vi "Dashboard2013.vi"() -> ()   [LabVIEW 2015]
uses:
  <vilib>/Utility/config.llb/NI_LVConfig.lvlib
  <vilib>/Utility/config.llb/Write Key (I32).vi
  globals/Angle.vi
  <vilib>/FTP/NI_FTP.lvlib
  <vilib>/vision/NI_Vision_Development_Module.lvlib
  <vilib>/Platform/browser.llb/Open URL in Default Browser (string).vi
  <vilib>/event_ctls.llb/eventvkey.ctl
  <vilib>/Utility/config.llb/Write Key (String).vi
  <vilib>/Utility/config.llb/Read Key (Double).vi
  <vilib>/Utility/config.llb/Write Key (Double).vi
  typeDefs/targetVariables.ctl
panel:
  in  "Filename":string="filename"
  in  "CaptureScreen":bool caption="OK Button"
  out "standard output":string
  in  "Tab Control":enum32{"Main", "Diagnostic"}(tab)
  in  "Viewer":enum32{"Camera", "Variables", "Files", "Misc"}(tab)
  out "Shoot Adjust":i8(slide) scale=-100.0..100.0 scale format="%4d"
  out "Image Error Message":string="Timeout in Camera Communications"
  out "Speed":cluster{dbl, dbl}(knob)={0.0, 3409.0831639982152} scale=2500.0..4300.0
  out "Frisbees":i16 format="%1.0f"
  out "Angle to Center":dbl format="%#_3g"
  out "Range to Center":dbl format="%-#3_3g"
  in  "Low Camera Settings":T1={"Frate Rate"=30, "Compression"=30, "Size"=1} {"Frate Rate" scale=1.0..30.0; "Size" items=["640x480", "320x240", "160x120"]}
  out "L Mbps":dbl format="%#.1g"
  in  "Low Cam Conf":bool
  out "BW":bool
  out "L_FPS":dbl format="%#.1g"
  out "Low Camera Image":T2(plugin-control) caption="Camera Image"
  in  "High Cam Conf":bool
  out "In Range":bool=TRUE
  out "Pre Hopper Time":dbl
  out "Pre-Jam":bool
  out "Batt Voltage":dbl
  in  "y":bool
  out "Tree":string(tree)
  in  "Open Auto Commands Doc":bool
  in  "Edit Vision Distance Table CSV":bool
  in  "Edit Autonomous CSV":bool
  in  "Transfer Vision Distance Table  to cRIO":bool
  in  "working directory":path=path "C:/BB/2013/Programming/Beachbot2013Dashboard"
  out "standard output":string
  in  "Transfer Autonomous CSV to cRIO":bool
  in  "Transfer INI From cRIO":bool
  in  "upper limit":dbl=20.0
  in  "lower limit":dbl=19.0
  in  "Dashboard Tab":T3(tab)
  in  "AutoWait":u16 caption="Autonomous Delay (Seconds)" format="%#7.0f"
  out "Battery Value":dbl(slide) scale=0.0..14.0 scale format="%#_2e"
  out "Battery":sgl(graph)
  out "Robot IP":string
  in  "Autonomous\nMode":u16(ring)
  in  "Number":dbl caption="rightDriveP"
  in  "Preferences Tree":string(tree)
  in  "Save":bool
  in  "On/Off":bool caption="~S A V E~"
  in  "String":string caption="Strings"
  in  "Slider":dbl(slide) scale=0.0..100.0 scale format="%#_3g"
  in  "What is this?":bool
  in  "Test Name":u16(ring) items=["Select the test to run...", "Example Test", "-------------------------------", "List of tests is built in robot code.", "Replace with your own automated tests."]
  in  "Test Tree":string(tree)
  in  "Motor":cluster{"Value":dbl, "Enable":bool} {"Value" scale=-1.0..1.0 scale format="%#_3g"}
  out "Progress":T4 {"Test Progress" scale=0.0..100.0}
  in  "Rev/Fwd":cluster{"Forward":bool, "Reverse":bool}
  in  "Ring":u16(ring) items=["Auto", "Fixed indoor", "Fixed outdoor 1", "Fixed outdoor 2", "Fixed fluorescent 1", "Fixed fluorescent 2", "Hold current"]
  in  "Listbox":i32(listbox)
  in  "BCG Low":T5={"Brightness"=212.0, "Contrast"=59.7, "Gamma"=0.64}
  out "Mode":T6(ring)=enum."Auto Disabled"
  in  "Alignment":i32=50
  in  "Targeting":i32=37
  out "Low Camera IP":string
  out "Target Info":T7(array[cluster]) {"Center Position"."X" format="%#_3g"; "Center Position"."Y" format="%#_3g"}
  in  "Camera view angle":dbl[](array[numeric])=[48.0, 43.5]
  out "Processed Image":T2(plugin-control)
  in  "Low Dilate_its":i32=11
  in  "Low Erode_its":i32=12
  in  "Low Brightness":i32=50
  out "Values":T8
  in  "Manual Video IP":bool
  out "Camera Image Diag":T2(plugin-control) caption="Camera Image"
  # "Shooting Range Setting"
  # "Audio Settings"
  # "Robot IP:"
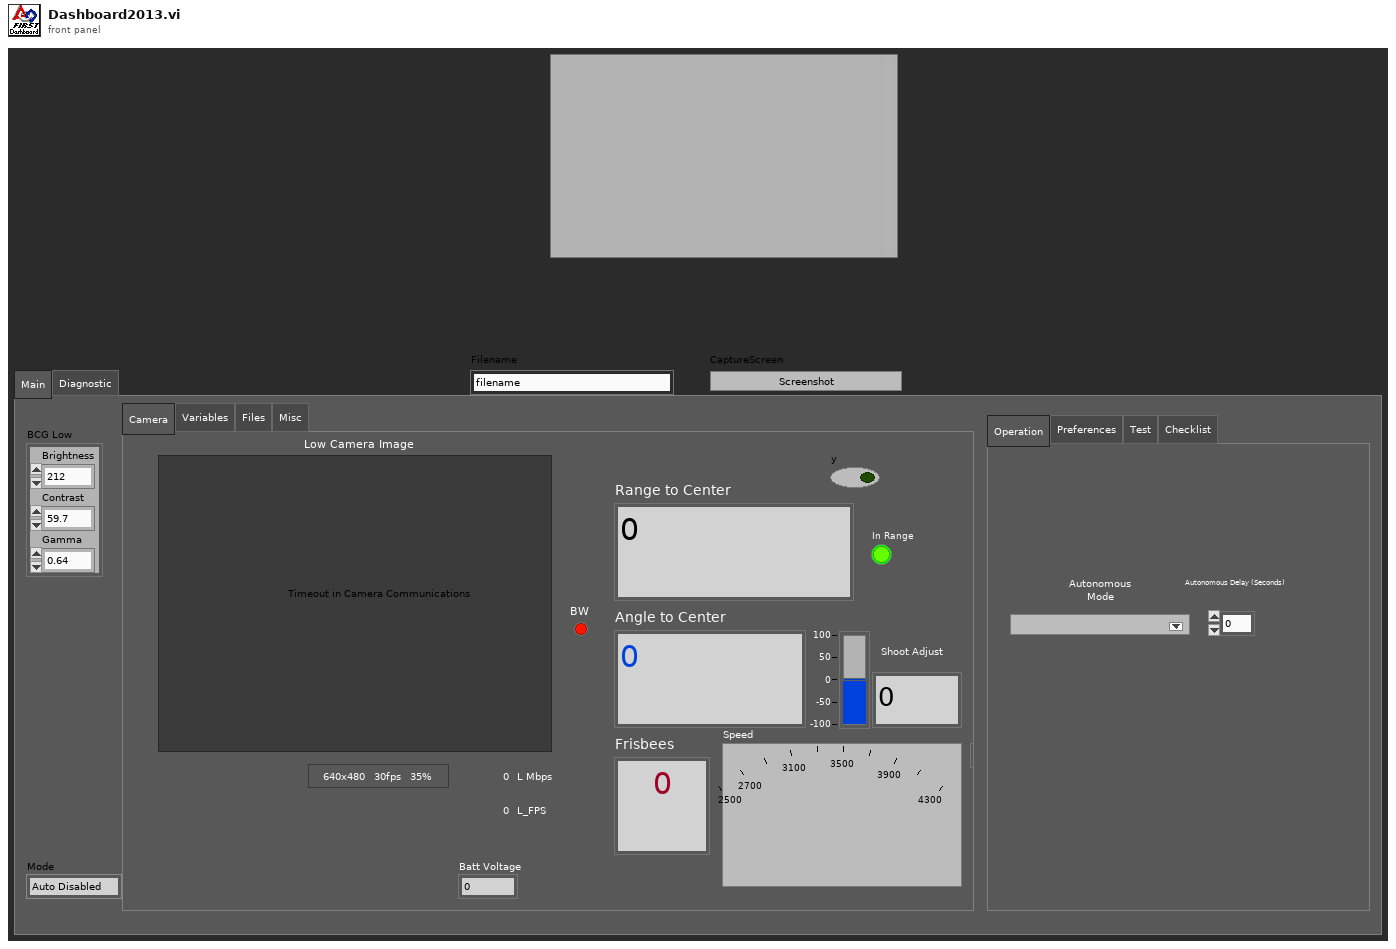
[diagram p1: front panel]
types:
  T1 = cluster{"Frate Rate":i32, "Compression":i32, "Size":u16}
  T2 = typedef "IMAQ Image.ctl" = refnum<image>
  T3 = enum32{"Operation", "Preferences", "Test", "Checklist"}
  T4 = cluster{"Test Progress":u8, "Test Progress Text":string}
  T5 = cluster{"Brightness":sgl, "Contrast":sgl, "Gamma":sgl}
  T6 = enum8{"Tele-Op Disabled", "Tele-Op Enabled", "Auto Disabled", "Auto Enabled", "Test Disabled", "Test Enabled", ""}
  T7 = cluster{"Center Position":cluster{"X":dbl, "Y":dbl}, "Distance":dbl, "targetType":enum16{"Center", "Side", "Vertical"}}[]
  T8 = typedef "targetVariables.ctl" = cluster{"distanceToCenter":dbl, "angleToCenter":dbl, "angleToLeft":dbl, "distanceToLeft":dbl, "angleToRight":dbl, "distanceToRight":dbl, "centerAge":dbl, "leftAge":dbl, "rightAge":dbl}
  T9 = typedef "Image Type" = u32
  T10 = typedef "Sound Output Task ID.ctl" = u32
  T11 = typedef "SkeletonTrackState.ctl" = enum32{"NotTracked", "PositionOnly", "Tracked"}
  T12 = cluster{"TrackingState":u8[], "Position":cluster{"x":sgl, "y":sgl, "z":sgl}, cluster{"x":sgl, "y":sgl, "z":sgl, sgl}[], "TrackState":T11}
  T13 = cluster{cluster{"ScaledToPercentRange":dbl, "ScaledToPercentRange":dbl, "ScaledToPercentRange":dbl}, cluster{bool, bool, bool}}[]
  T14 = cluster{cluster{"ScaledToPercentRange":dbl, "ScaledToPercentRange":dbl, "ScaledToPercentRange":dbl}, cluster{bool, bool, bool}}
  T15 = typedef "LVRectTypeDef.ctl" = cluster{"Left":i16, "Top":i16, "Right":i16, "Bottom":i16}
  T16 = cluster{"Competition mode":bool, "Robot Link":bool, "Autonomous":bool, "Enabled":bool, "E-Stop":bool, "Simulated":bool, "TestMode":bool, "Docked Window":bool}
  T17 = typedef "NI_LVConfig.lvlib/Config Data RefNum.ctl" = refnum<k1>
  T18 = typedef "eventvkey.ctl" = enum16{"ASCII", "Enter", "Return", "Shift", "Ctrl", "Alt", "Cmd", "Opt", "Caps", "NumLock", "Clear", "Break", "Up", "Down", "Left", "Right", "Insert", "Delete", "Home", "End", "PageUp", "PageDown", "Escape", "Help", "Pause", "ScrollLock", "F1", "F2", "F3", "F4", "F5", "F6", "F7", "F8", "F9", "F10", "F11", "F12", "F13", "F14", "F15", "F16", "F17", "F18", "F19", "F20", "F21", "F22", "F23", "F24", "Play", "VolumeUp", "VolumeDown", "Mute", "Two Byte Char"}
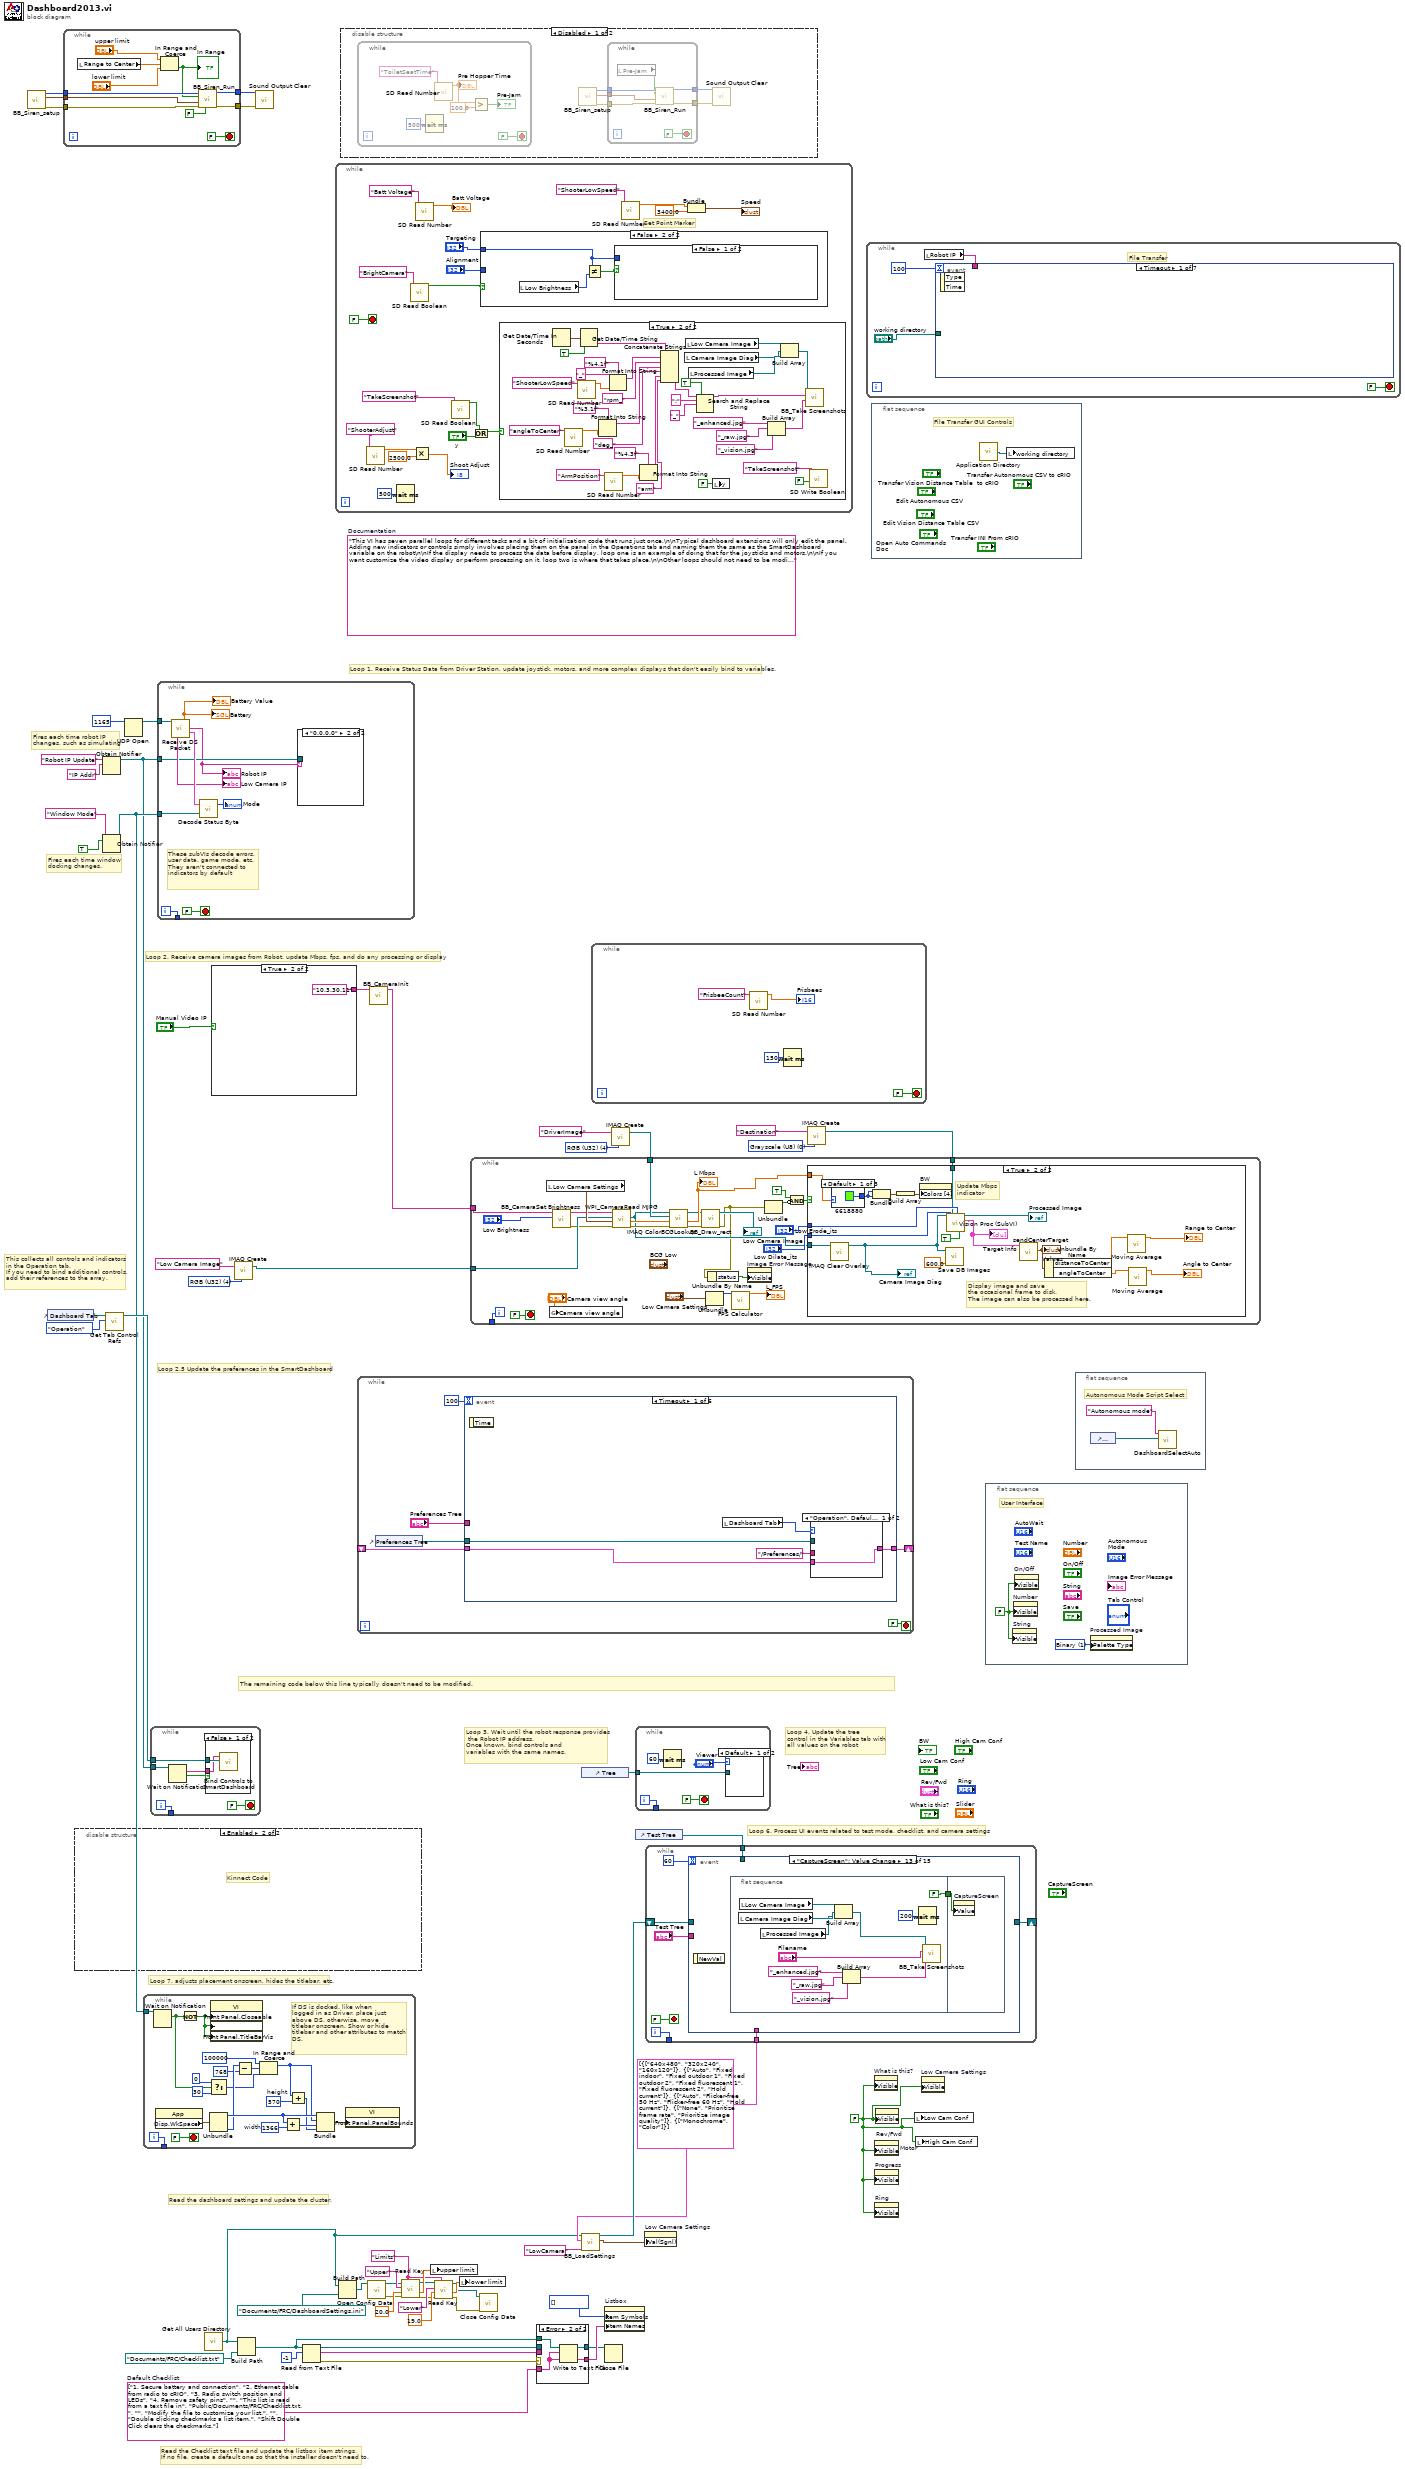
[diagram p0: block diagram]
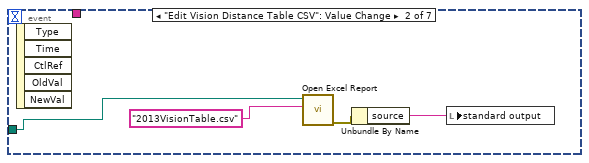
[diagram p2: hidden frame]
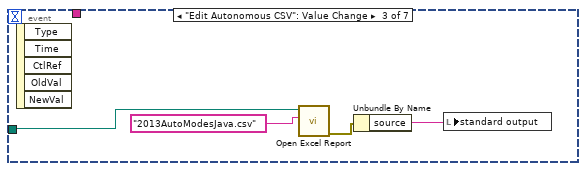
[diagram p3: hidden frame]
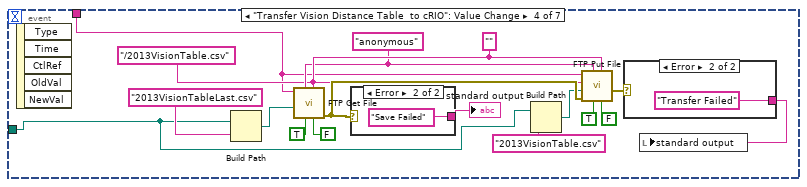
[diagram p4: hidden frame]
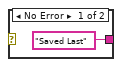
[diagram p5: hidden frame]
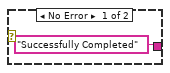
[diagram p6: hidden frame]
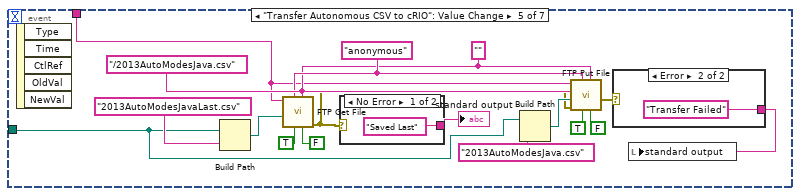
[diagram p7: hidden frame]
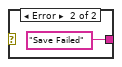
[diagram p8: hidden frame]
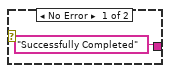
[diagram p9: hidden frame]
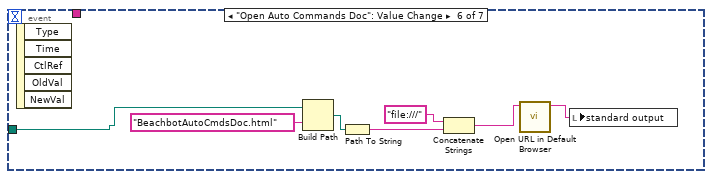
[diagram p10: hidden frame]
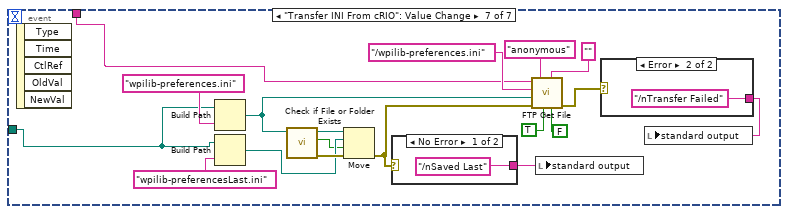
[diagram p11: hidden frame]
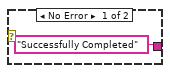
[diagram p12: hidden frame]
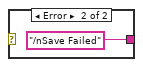
[diagram p13: hidden frame]
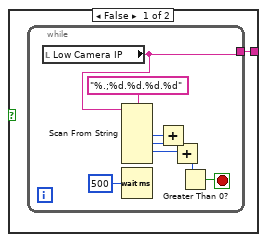
[diagram p15: hidden frame]
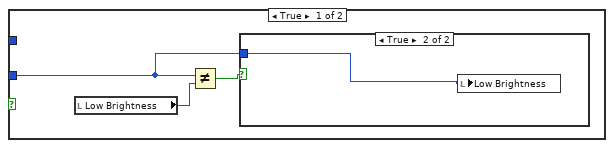
[diagram p16: hidden frame]
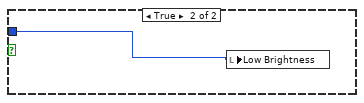
[diagram p18: hidden frame]
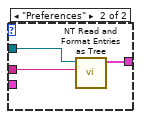
[diagram p20: hidden frame]
diagram:
  w8 = "Limits" ("section")
  w24 = T9 4 items=["Grayscale (U8)", "Grayscale (I16)", "Grayscale (SGL)", "Complex (CSG)", "RGB (U32)", "HSL (U32)", "RGB (U64)"] ("Image Type")
  w31 = T9 0 items=["Grayscale (U8)", "Grayscale (I16)", "Grayscale (SGL)", "Complex (CSG)", "RGB (U32)", "HSL (U32)", "RGB (U64)"] ("Image Type")
  w37 = T9 4 items=["Grayscale (U8)", "Grayscale (I16)", "Grayscale (SGL)", "Complex (CSG)", "RGB (U32)", "HSL (U32)", "RGB (U64)"] ("Image Type")
  w33 = cluster{string[]}[] [{["640x480", "320x240", "160x120"]}, {["Auto", "Fixed indoor", "Fixed outdoor 1", "Fixed outdoor 2", "Fixed fluorescent 1", "Fixed fluorescent 2", "Hold current"]}, {["Auto", "Flicker-free 50 Hz", "Flicker-free 60 Hz", "Hold current"]}, {["None", "Prioritize frame rate", "Prioritize image quality"]}, {["Monochrome", "Color"]}]
  w45 = string[] ["1. Secure battery and connection", "2. Ethernet cable from radio to cRIO", "3. Radio switch position and LEDs", "4. Remove safety pins", "", "This list is read from a text file in", "Public/Documents/FRC/Checklist.txt.", "", "Modify the file to customize your list.", "", "Double clicking checkmarks a list item.", "Shift Double Click clears the checkmarks."]  # Default Checklist
  w32 = FALSE ("Visible")
  (unwired) "This VI has seven parallel loops for different tasks and a bit of initialization code that runs just once.\n\nTypical dashboard extensions will only edit the panel. Adding new indicators or controls simply involves placing them on the panel in the Operations tab and naming them the same as the SmartDashboard variable on the robot\n\nIf the display needs to process the data before display, loop one is an example of doing that for the joysticks and motors.\n\nIf you want customize the video display or perform processing on it, loop two is where that takes place.\n\nOther loops should not need to be modified. They are pretty standard, and document the task they perform."  # Documentation
  # "Loop 2.5 Update the preferences in the SmartDashboard"
  # "Fires each time robot IP\nchanges, such as simulating"
  # "Fires each time window\ndocking changes."
  # "Read the Checklist text file and update the listbox item strings.\nIf no file, create a default one so that the installer doesn't need to."
  # "This collects all controls and indicators\nin the Operation tab.\nIf you need to bind additional controls,\nadd their references to the array."
  # "The remaining code below this line typically doesn't need to be modified."
  # "Loop 6. Process UI events related to test mode, checklist, and camera settings"
  # "Read the dashboard settings and update the cluster."
  # "Loop 4. Update the tree\ncontrol in the Variables tab with\nall values on the robot"
  # "Loop 3. Wait until the robot response provides\n the Robot IP address.\nOnce known, bind controls and\nvariables with the same names."
  # "Loop 7. adjusts placement onscreen, hides the titlebar, etc."
  # "Loop 1. Receive Status Data from Driver Station, update joystick, motors, and more complex displays that don't easily bind to variables."
  # "Loop 2. Receive camera images from Robot, update Mbps, fps, and do any processing or display"
  n1 = call "BB_Siren_setup.vi"() -> ("error out"=w20:errorcluster, "Sampling Info"=w19:cluster{"Fs":dbl, "#s":dbl}, "task ID"=w21:T10)  [unwired: 9 in]
  n2 = control-ref of="Dashboard Tab"() -> (w58:refnum<vi>)
  n3 = while {
    tunnel: w21 -> [w71]
    tunnel: w20 -> [w70]
    tunnel: w19 -> [w69]
    tunnel: [w68] -> w18
    tunnel: [w67] -> w17
    stop <- FALSE stop-if-true
    n4 = local read "Range to Center"() -> (w66:dbl)
    n5 = In Range and Coerce(upper limit="upper limit", x=w66, lower limit="lower limit") -> (In Range?=w65:bool)  [unwired: 1 out]
    "In Range" <- w65
    n6 = call "BB_Siren_Run.vi"("Oscillate"=FALSE, "Error In"=w70, "sampling info"=w69, "Active"=w65, "Task ID In"=w71) -> ("error out"=w68:errorcluster, "task ID out"=w67:T10)  [unwired: 5 in]
  }
  n7 = disable-structure shown="Enabled" {
    frame Disabled {
      # "Loop 5. Receive Kinect data from Driver Station and update visualization"
      n8 = UDP Open(11:u16 1166 ("port")) -> (port=w73:refnum<k16>)  [unwired: 2 in, 4 out]
      n9 = while {
        tunnel: w73 -> [w83]
        tunnel: [w76] -> _
        i -> [w76]
        stop <- FALSE stop-if-true
        n10 = UDP Read(connection ID=w83, max size (548)=1018 ("bytes to read"), timeout ms (25000)=1000) -> (data out=w81:string, error out=w75:errorcluster)  [unwired: 1 in, 3 out]
        n11 = call "Build Simple Skeleton Data.vi"("error in (no error)"=w75, "data in"=w81) -> ("Skeleton Data"=w82:T12, "Simple Joystick Info"=w79:T13)  [unwired: 5 in, 3 out]
        n12 = call "Draw Simple Skeleton Picture.vi"("Simple Skeleton"=w82) -> ()  [unwired: 10 in, 1 out]
        n13 = Index Array(array=w79) -> (element #1=w78:T14, element #2=w77:T14)  [unwired: 2 in]
        n14 = Unbundle(w78) -> ()  [unwired: 2 out]
        n15 = Unbundle(w77) -> ()  [unwired: 2 out]
      }
    }
    frame Enabled {
      # "Kinnect Code"
    }
  }
  n16 = Obtain Notifier(name (unnamed)="Robot IP Update", notification data type="IP Addr" ("name (unnamed)")) -> (notifier out=w22:refnum<notifier>)  [unwired: 2 in, 2 out]
  n17 = Obtain Notifier(name (unnamed)="Window Mode", notification data type=TRUE) -> (notifier out=w49:refnum<notifier>)  [unwired: 2 in, 2 out]
  n18 = call <vilib>:"Get Tab Control Refs.vi"("Page Index"=enum32{"Operation", "Test"}."Operation" ("Dashboard Tab"), "TabControl in"=w58) -> ("ControlsOnPage"=w59:refnum<vi>[])  [unwired: 9 in]
  n19 = UDP Open(11:u16 1165 ("port")) -> (port=w60:refnum<k16>)  [unwired: 2 in, 4 out]
  n20 = while {
    tunnel: w49 -> [w104]
    tunnel: [w102] -> _
    i -> [w102]
    stop <- FALSE stop-if-true
    w94 = 1366  # width
    w97 = 570  # height
    # "If DS is docked, like when\nlogged in as Driver, place just\nabove DS, otherwise, move\ntitlebar onscreen. Show or hide\ntitlebar and other attributes to match\nDS."
    n21 = Wait on Notification(notifier=w104) -> (notification=w89:bool)  [unwired: 3 in, 3 out]
    n22 = property class="App"() -> ("Disp.WkSpace"=w100:T15)  [unwired: 2 in, 2 out]
    n23 = Not(x=w89) -> (.not. x?=w103:bool)
    n24 = Unbundle(w100) -> ("Left"=w98:i16, "Bottom"=w95:i16)  [unwired: 2 out]
    n25 = Select(t=0, s=w89, f=30) -> (s? t:f=w88:i32)
    n26 = property class="VI"("Front Panel.Closeable"=w103, "Front Panel.Minimizeable"=w103, "Front Panel.TitleBarVis"=w103) -> ()  [unwired: 2 in, 2 out]
    n27 = Subtract(x=w95, y=768) -> (x-y=w92:i32)
    n28 = In Range and Coerce(upper limit=100000, x=w92, lower limit=w88) -> (coerced(x)=w86:i32)  [unwired: 1 out]
    n29 = Add(x=w98, y=w94) -> (x+y=w99:i32)
    n30 = Add(x=w86, y=w97) -> (x+y=w96:i32)
    n31 = Bundle("Left"=w98, w86, w99, w96) -> (w101:cluster{"Left":i16, i32, i32, i32})  [unwired: 1 out]
    n32 = property class="VI"("Front Panel.PanelBounds"=w101) -> ()  [unwired: 2 in, 2 out]
  }
  n33 = while {
    tunnel: w59 -> [w111]
    tunnel: w22 -> [w108]
    tunnel: [w106] -> _
    i -> [w106]
    stop <- FALSE stop-if-true
    n34 = Wait on Notification(notifier=w108) -> (notification=w107:string, timed out?=w109:bool)  [unwired: 3 in, 2 out]
    n35 = case shown="False" w109 {
      tunnel: w111 -> [w113 _]
      tunnel: w107 -> [w112 _]
      frame False {
        n36 = call <vilib>:"Bind Controls to SmartDashboard.vi"("Bound Control Refs"=w113, "Server IP Address"=w112) -> ()  [unwired: 10 in]
      }
      frame True {
      }
    }
  }
  n37 = while {
    tunnel: w60 -> [w121]
    tunnel: w49 -> [w119]
    tunnel: [w116] -> _
    tunnel: w22 -> [w115]
    i -> [w116]
    stop <- FALSE stop-if-true
    # "These subVIs decode errors, user data, game mode, etc.\nThey aren't connected to indicators by default"
    n38 = call "Receive DS Packet.vi"("Recv Socket"=w121) -> ("Battery"=→"Battery" →"Battery Value":sgl, "Robot IP Address"=w114:string, "Status"=w122:T16, "Low Camera IP Address"=→"Low Camera IP":string)  [unwired: 1 in, 10 out]
    "Robot IP" <- w114
    n39 = call "Decode Status Byte.vi"("Window Mode Notifier"=w119, "Status"=w122) -> ("Mode"=→"Mode":T6)  [unwired: 1 out]
    n40 = case shown="\"0.0.0.0\"" w114 {
      selector: w114 -> [w124 _]
      tunnel: w115 -> [w125 _]
      frame Default {
        n41 = Send Notification(notification=w124, notifier=w125) -> ()  [unwired: 1 in, 2 out]
      }
      frame "0.0.0.0" {
      }
    }
  }
  n42 = call "Get All Users Directory.vi"() -> ("All User Path"=w13:path)
  n43 = case shown="True" "Manual Video IP" {
    tunnel: [w126 "10.3.30.11" ("Low Camera IP")] -> w35
    frame False {
      n44 = while {
        tunnel: [w128] -> w126
        stop <- w127 stop-if-true
        n45 = local read "Low Camera IP"() -> (w128:string)
        n46 = Scan From String(format string="%.;%d.%d.%d.%d", input string=w128) -> (output 1=w133:i32, output 2=w134:i32, output 3=w131:i32)  [unwired: 2 in, 8 out]
        n47 = Wait (ms)(milliseconds to wait=u32 500) -> ()  [unwired: 1 out]
        n48 = Add(x=w133, y=w134) -> (x+y=w132:i32)
        n49 = Add(x=w132, y=w131) -> (x+y=w130:i32)
        n50 = Greater Than 0?(x=w130) -> (x > 0?=w127:bool)
      }
    }
    frame True {
    }
  }
  n51 = call "IMAQ Create"("Image Name"="Low Camera Image", "Image Type"=w37) -> ("New Image"=w26:T2)  [unwired: 2 in, 2 out]
  n52 = Build Path(base path=w13, name or relative path=path "Documents/FRC/Checklist.txt") -> (appended path=w46:path)
  n53 = call <vilib>:"Sound Output Clear.vi"("error in (no error)"=w18, "task ID"=w17) -> ()  [unwired: 9 in, 1 out]
  n54 = Read from Text File(file (use dialog)=w46, count=-1 ("timeout ms (25000)")) -> (refnum out=w43:refnum<file>, text=w47:string[], error out=w48:errorcluster)  [unwired: 2 in, 1 out]
  n55 = while {
    stop <- FALSE stop-if-true
    # "Set Point Marker"
    n56 = call <vilib>:"SD Read Number.vi"("Name"="ShooterAdjust") -> ("Numeric"=w142:dbl)  [unwired: 8 in, 2 out]
    n57 = Wait (ms)(milliseconds to wait=u32 500) -> ()  [unwired: 1 out]
    n58 = call <vilib>:"SD Read Boolean.vi"("Name"="BrightCamera") -> ("Boolean"=w153:bool)  [unwired: 8 in, 2 out]
    n59 = Multiply(x=w142, y=2500.0) -> (x*y=→"Shoot Adjust":dbl)
    n60 = call <vilib>:"SD Read Number.vi"("Name"="Batt Voltage") -> ("Numeric"=→"Batt Voltage":dbl)  [unwired: 8 in, 2 out]
    n61 = call <vilib>:"SD Read Boolean.vi"("Name"="TakeScreenshot") -> ("Boolean"=w139:bool)  [unwired: 8 in, 2 out]
    n62 = Or(x=w139, y="y") -> (x .or. y?=w138:bool)
    n63 = case shown="False" w153 {
      tunnel: "Targeting" -> [_ w161]
      tunnel: "Alignment" -> [w157 _]
      frame True {
        n64 = local read "Low Brightness"() -> (w159:i32)
        n65 = Not Equal?(x=w157, y=w159) -> (x != y?=w158:bool)
        n66 = case shown="True" w158 {
          tunnel: w157 -> [_ w160]
          frame False {
          }
          frame True {
            n67 = local write "Low Brightness"(w160) -> ()
          }
        }
      }
      frame False {
        n68 = local read "Low Brightness"() -> (w163:i32)
        n69 = Not Equal?(x=w161, y=w163) -> (x != y?=w162:bool)
        n70 = case shown="False" w162 {
          tunnel: w161 -> [_ w164]
          frame False {
          }
          frame True {
            n71 = local write "Low Brightness"(w164) -> ()
          }
        }
      }
    }
    n72 = case shown="True" w138 {
      frame False {
      }
      frame True {
        n73 = Get Date/Time In Seconds() -> (seconds since 1Jan1904=w197:timestamp)
        n74 = call <vilib>:"SD Read Number.vi"("Name"="angleToCenter") -> ("Numeric"=w188:dbl)  [unwired: 8 in, 2 out]
        n75 = call <vilib>:"SD Read Number.vi"("Name"="ShooterLowSpeed") -> ("Numeric"=w194:dbl)  [unwired: 8 in, 2 out]
        n76 = Get Date/Time String(seconds (now)=w197, want seconds? (F)=TRUE) -> (time string=w195:string)  [unwired: 1 in, 1 out]
        n77 = Format Into String(format string="%3.1f", w188) -> (resulting string=w187:string)  [unwired: 2 in, 1 out]
        n78 = call <vilib>:"SD Read Number.vi"("Name"="ArmPosition") -> ("Numeric"=w170:dbl)  [unwired: 8 in, 2 out]
        n79 = Format Into String(format string="%4.1f", initial string="_", w194) -> (resulting string=w191:string)  [unwired: 1 in, 1 out]
        n80 = Format Into String(format string="%4.3f", w170) -> (resulting string=w167:string)  [unwired: 2 in, 1 out]
        n81 = Concatenate Strings(w195, w191, "rpm_", w187, "deg_" ("string"), w167, "arm" ("string")) -> (w174:string)
        n82 = local read "Camera Image Diag"() -> (w180:T2)
        n83 = local read "Low Camera Image"() -> (w179:T2)
        n84 = local read "Processed Image"() -> (w181:T2)
        n85 = Search and Replace String(replace all?=TRUE ("replace all? (F)"), input string=w174, search string=":", replace string="_" ("replace string (\"\")")) -> (result string=w175:string)  [unwired: 4 in, 3 out]
        n86 = local write "y"(FALSE ("y")) -> ()
        n87 = Build Array("_enhanced.jpg", "_raw.jpg", "_vision.jpg") -> (w182:string[])
        n88 = Build Array(w179, w180, w181) -> (w178:T2[])
        n89 = call "BB_Take Screenshots.vi"("Image_Labels"=w182, "Prefix"=w175, "Image_Array"=w178) -> ()  [unwired: 8 in, 1 out]
        n90 = call <vilib>:"SD Write Boolean.vi"("Boolean"=FALSE, "Name"="TakeScreenshot") -> ()  [unwired: 8 in, 2 out]
      }
    }
    n91 = call <vilib>:"SD Read Number.vi"("Name"="ShooterLowSpeed") -> ("Numeric"=w148:dbl)  [unwired: 8 in, 2 out]
    n92 = Bundle("Numeric"=w148, "element"=3400.0) -> (→"Speed":cluster{"Numeric":dbl, "element":dbl})  [unwired: 1 in]
  }
  n93 = Build Path(base path=w13, name or relative path=path "Documents/FRC/DashboardSettings.ini") -> (appended path=w14:path)
  n94 = disable-structure shown="Disabled" {
    frame Disabled {
      n95 = while {
        stop <- FALSE stop-if-true
        n96 = Wait (ms)(milliseconds to wait=u32 500) -> ()  [unwired: 1 out]
        n97 = call <vilib>:"SD Read Number.vi"("Name"="ToiletSeatTime") -> ("Numeric"=w208:dbl)  [unwired: 8 in, 2 out]
        "Pre Hopper Time" <- w208
        n98 = Greater?(x=w208, y=100.0) -> (0:→"Pre-Jam":bool)
      }
      n99 = call "BB_Siren_setup.vi"() -> ("error out"=w203:errorcluster, "Sampling Info"=w202:cluster{"Fs":dbl, "#s":dbl}, "task ID"=w204:T10)  [unwired: 9 in]
      n100 = while {
        tunnel: w204 -> [w216]
        tunnel: w203 -> [w215]
        tunnel: w202 -> [w214]
        tunnel: [w213] -> w201
        tunnel: [w212] -> w200
        stop <- FALSE stop-if-true
        n101 = local read "Pre-Jam"() -> (w211:bool)
        n102 = call "BB_Siren_Run.vi"("Error In"=w215, "sampling info"=w214, "Active"=w211, "Task ID In"=w216) -> ("error out"=w213:errorcluster, "task ID out"=w212:T10)  [unwired: 6 in]
      }
      n103 = call <vilib>:"Sound Output Clear.vi"("error in (no error)"=w201, "task ID"=w200) -> ()  [unwired: 9 in, 1 out]
    }
    frame Enabled {
    }
  }
  n104 = while {
    shift-right: [w219] -> _
    shift-left: _ -> [w218]
    stop <- FALSE stop-if-true
    n105 = control-ref of="Preferences Tree"() -> (w221:refnum<vi>)
    n106 = event shown="[0] Timeout" {
      selector: _ -> [_ _ _ _ _ _]
      dyn-events: _ -> [_ _ _ _ _ _]
      timeout: u32 100 ("milliseconds to wait") -> [_ _ _ _ _ _]
      tunnel: w221 -> [w226 w239 _ _ _ _]
      tunnel: "Preferences Tree" -> [_ _ w260 w266 w268 _]
      tunnel: [w227 w233 w259 w265 w267 w270] -> w219
      tunnel: w218 -> [w225 w233 w259 w265 w267 w270]
      event Timeout {
        n107 = event-data() -> ()  [unwired: 1 in, 1 out]
        n108 = local read "Dashboard Tab"() -> (w224:T3)
        n109 = case shown="\"Operation\", Default" w224 {
          tunnel: w226 -> [_ w232]
          tunnel: "/Preferences/" ("Name Pattern") -> [_ w231]
          tunnel: [w229 w230] -> w227
          tunnel: w225 -> [w229 _]
          frame "Operation", Default {
          }
          frame "Preferences" {
            n110 = call <vilib>:"NT Read and Format Entries as Tree.vi"("Name Pattern"=w231, "Tree Refnum"=w232) -> ("Formatted Strings"=w230:cluster{"Name":string, "Value":string}[])  [unwired: 8 in, 1 out]
          }
        }
      }
      event "Preferences Tree": Value Change {
        # "Remove Prefix"
        n111 = event-data() -> ("NewVal"=w237:string)  [unwired: 1 in, 1 out]
        n112 = for {
          tunnel: w233 -> [w245] mode=indexing
          tunnel: w237 -> [w244]
          tunnel: [w242] -> w238
          tunnel: [w241] -> w236
          stop <- w243 stop-if-true
          # "Find value for name"
          n113 = Unbundle By Name(w245) -> ("Name"=w241:string, "Value"=w242:string)
          n114 = Equal?(x=w241, y=w244) -> (x = y?=w243:bool)
        }
        n115 = call "DecodeNTType.vi"("string"=w238) -> ("type"=w240:string)  [unwired: 7 in, 3 out]
        n116 = String Subset(string=w236, offset (0)=13) -> (substring=w235:string)  [unwired: 1 in]
        n117 = case shown="Default" w240 {
          tunnel: w239 -> [_ _ _ _]
          tunnel: w235 -> [_ w247 w250 w254]
          frame Default {
            w246 = FALSE ("Visible")
            n118 = property on="String" class="Str"("Visible"=w246) -> ()  [unwired: 2 in, 2 out]
            n119 = property on="On/Off" class="Bool (strict)"("Visible"=w246) -> ()  [unwired: 2 in, 2 out]
            n120 = property on="Number" class="DigNum (strict)"("Visible"=w246) -> ()  [unwired: 2 in, 2 out]
          }
          frame "Number" {
            w248 = FALSE ("Visible")
            n121 = property on="On/Off" class="Bool (strict)"("Visible"=w248) -> ()  [unwired: 2 in, 2 out]
            n122 = property on="String" class="Str"("Visible"=w248) -> ()  [unwired: 2 in, 2 out]
            n123 = property on="Number" class="DigNum (strict)"("Visible"=TRUE, "Caption.Text"=w247) -> ()  [unwired: 2 in, 2 out]
          }
          frame "String" {
            w251 = FALSE ("Visible")
            n124 = property on="Number" class="DigNum (strict)"("Visible"=w251) -> ()  [unwired: 2 in, 2 out]
            n125 = property on="On/Off" class="Bool (strict)"("Visible"=w251) -> ()  [unwired: 2 in, 2 out]
            n126 = property on="String" class="Str"("Visible"=TRUE, "Caption.Text"=w250) -> ()  [unwired: 2 in, 2 out]
          }
          frame "Boolean" {
            w253 = FALSE ("Visible")
            # "Get direction and finish"
            n127 = property on="String" class="Str"("Visible"=w253) -> ()  [unwired: 2 in, 2 out]
            n128 = property on="Number" class="DigNum (strict)"("Visible"=w253) -> ()  [unwired: 2 in, 2 out]
            n129 = property on="On/Off" class="Bool (strict)"("Visible"=TRUE, "Caption.Text"=w254) -> ()  [unwired: 2 in, 2 out]
          }
        }
      }
      event "Number": Value Change {
        n130 = event-data() -> ("NewVal"=w258:dbl)  [unwired: 1 in]
        n131 = Format Value(format string="%.3f", value (0)=w258) -> (output string=w256:string)  [unwired: 1 in]
        n132 = call <vilib>:"NT Write String.vi"("String"=w256, "Name"=w260) -> ()  [unwired: 9 in, 1 out]
      }
      event "On/Off": Value Change {
        n133 = event-data() -> ("NewVal"=w264:bool)  [unwired: 1 in]
        n134 = Select(t="True", s=w264, f="False") -> (s? t:f=w261:string)
        n135 = call <vilib>:"NT Write String.vi"("String"=w261, "Name"=w266) -> ()  [unwired: 9 in, 1 out]
      }
      event "String": Value Change {
        n136 = event-data() -> ("NewVal"=w269:string)  [unwired: 1 in]
        n137 = call <vilib>:"NT Write String.vi"("String"=w269, "Name"=w268) -> ()  [unwired: 9 in, 1 out]
      }
      event "Save": Value Change {
        n138 = event-data() -> ("NewVal"=w272:bool)  [unwired: 1 in]
        n139 = call <vilib>:"NT Write Boolean.vi"("Boolean"=w272, "Name"="/Preferences/~S A V E~") -> ()  [unwired: 9 in, 1 out]
      }
    }
  }
  n140 = call <vilib>:"Open Config Data.vi"("configuration file path"=w14) -> ("error out"=w4:errorcluster, "refnum"=w9:T17)  [unwired: 8 in, 1 out]
  n141 = call "BB_CameraInit.vi"("Camera IP In"=w35) -> ("Camera IP Out"=w27:string)  [unwired: 10 in]
  n142 = call-poly <vilib>:"Read Key.vi"("section"=w8, "error in (no error)"=w4, "default value"=20.0, "key"="Upper", "refnum"=w9) -> ("error out"=w5:errorcluster, "value"=w11:dbl, "refnum out"=w10:T17)  [unwired: 4 out]
  n143 = local write "upper limit"(w11) -> ()
  n144 = call-poly <vilib>:"Read Key.vi"("section"=w8, "error in (no error)"=w5, "default value"=19.0, "key"="Lower", "refnum"=w10) -> ("error out"=w1:errorcluster, "value"=w3:dbl, "refnum out"=w2:T17)  [unwired: 4 out]
  n145 = local write "lower limit"(w3) -> ()
  n146 = call <vilib>:"Close Config Data.vi"("error in (no error)"=w1, "refnum"=w2) -> ()  [unwired: 1 in, 9 out]
  n147 = case shown="Error" w48 {
    tunnel: w47 -> [w274 _]
    tunnel: [w274 w276] -> w44
    tunnel: w45 -> [_ w276]
    tunnel: w46 -> [_ w277]
    tunnel: [w273 w275] -> w42
    tunnel: w43 -> [w273 _]
    frame No Error {
    }
    frame Error {
      n148 = Write to Text File(file (use dialog)=w277, text=w276) -> (refnum out=w275:refnum<file>)  [unwired: 2 in, 2 out]
    }
  }
  n149 = call "BB_LoadSettings.vi"("Section"="LowCamera", "Array"=w33, "All User Path"=w13) -> ("Cluster"=w41:cluster{"value":i32, "value":i32, "index":i32}, "Refnum out"=w40:T17)  [unwired: 7 in]
  n150 = control-ref of="Tree"() -> (w39:refnum<vi>)
  n151 = while {
    stop <- FALSE stop-if-true
    n152 = call <vilib>:"SD Read Number.vi"("Name"="FrisbeeCount") -> ("Numeric"=→"Frisbees":dbl)  [unwired: 8 in, 2 out]
    n153 = Wait (ms)(milliseconds to wait=u32 150) -> ()  [unwired: 1 out]
  }
  n154 = property on="Listbox" class="LstBox (strict)"("Item Symbols"=i32[] [], "Item Names"=w44) -> ()  [unwired: 2 in, 2 out]
  n155 = Close File(refnum=w42) -> ()  [unwired: 1 in, 2 out]
  n156 = call "IMAQ Create"("Image Name"="DriverImage", "Image Type"=w24) -> ("New Image"=w23:T2)  [unwired: 2 in, 2 out]
  n157 = while {
    tunnel: [w283] -> _
    tunnel: w39 -> [w282]
    i -> [w283]
    stop <- FALSE stop-if-true
    n158 = Wait (ms)(milliseconds to wait=u32 60) -> ()  [unwired: 1 out]
    n159 = case shown="Default" "Viewer" {
      tunnel: w282 -> [_ w287]
      frame Default {
      }
      frame "Variables" {
        n160 = call <vilib>:"NT Read and Format Entries as Tree.vi"("Tree Refnum"=w287) -> ()  [unwired: 9 in, 2 out]
      }
    }
  }
  n161 = control-ref of="Test Tree"() -> (w38:refnum<vi>)
  n162 = property on="Low Camera Settings" class="Clust (strict)"("Val(Sgnl)"=w41) -> ()  [unwired: 2 in, 2 out]
  n163 = while {
    tunnel: w33 -> [w292]
    shift-right: [w291] -> _
    shift-left: w40 -> [w290]
    tunnel: [w289] -> _
    tunnel: w38 -> [w288]
    i -> [w289]
    stop <- FALSE stop-if-true
    n164 = event shown="[12] \"CaptureScreen\": Value Change" {
      selector: _ -> [_ _ _ _ _ _ _ _ _ _ _ _ _ _ _]
      dyn-events: _ -> [_ _ _ _ _ _ _ _ _ _ _ _ _ _ _]
      timeout: u32 60 ("milliseconds to wait") -> [_ _ _ _ _ _ _ _ _ _ _ _ _ _ _]
      tunnel: w288 -> [w302 _ _ _ _ _ _ _ _ _ _ _ _ _ _]
      tunnel: "Test Tree" -> [_ _ _ _ _ _ _ _ _ w506 w514 w516 _ w533 w541]
      tunnel: w292 -> [_ w324 _ _ _ _ w460 _ w500 _ _ _ _ _ _]
      tunnel: [w296 w323 _ w426 w434 w446 w459 w488 w493 w505 w512 w515 _ w532 w540] -> w291
      tunnel: w290 -> [w296 w323 _ w426 w434 w446 w458 w492 w493 w505 w512 w515 _ w532 w540]
      event Timeout {
        w301 = enum16{"Update", "Clear"}[] [enum."Clear", enum."Clear", enum."Clear", enum."Clear", enum."Update", enum."Update", enum."Clear"] items=["Update", "Clear"]
        n165 = event-data() -> ()  [unwired: 1 in, 1 out]
        n166 = local read "Mode"() -> (w299:T6)
        n167 = Index Array(array=w301, index=w299) -> (element=w300:enum16{"Update", "Clear"})
        n168 = call <vilib>:"NT Read String.vi"("Name"="TestMode/TestName") -> ("String"=w305:string)  [unwired: 9 in, 1 out]
        n169 = case shown="\"Operation\", Default" "Dashboard Tab" {
          tunnel: w302 -> [_ w315]
          tunnel: "/TestMode/Automatic/" ("Name Pattern") -> [_ w314]
          tunnel: w300 -> [_ w313]
          tunnel: w299 -> [_ w311]
          frame "Operation", Default {
          }
          frame "Test" {
            w310 = -2 ("Active Item:Row Number")
            n170 = call <vilib>:"NT Read and Format Entries as Tree.vi"("Operation"=w313, "Name Pattern"=w314, "Tree Refnum"=w315) -> ()  [unwired: 7 in, 2 out]
            n171 = Index Array(array=u32[] [14013909, 14013909, 14013909, 14013909, 14013909, 16777215, 14013909], index=w311) -> (element=w309:u32)
            n172 = property on="Test Tree" class="Tree (strict)"("Active Item Row Number"=w310, "ActiveColNum"=w310, "CellBG"=w309, "Active Item Row Number"=-1 ("Active Item:Row Number"), "CellBG"=u32 5789784 ("Color Box")) -> ()  [unwired: 2 in, 2 out]
          }
        }
        n173 = case shown="\"\"" w305 {
          tunnel: "TestMode/TestProgress" ("Name") -> [w317 _]
          tunnel: "TestMode/TestProgressText" ("Name") -> [w316 _]
          frame Default {
            n174 = call <vilib>:"NT Read Number.vi"("Name"=w317) -> ("Numeric"=w318:dbl)  [unwired: 9 in, 1 out]
            n175 = call <vilib>:"NT Read String.vi"("Name"=w316) -> ("String"=w319:string)  [unwired: 9 in, 1 out]
            n176 = Bundle("Numeric"=w318, "String"=w319) -> (→"Progress":cluster{"Numeric":dbl, "String":string})  [unwired: 1 in]
          }
          frame "" {
            n177 = property on="Progress" class="Clust (strict)"("Visible"=FALSE) -> ()  [unwired: 2 in, 2 out]
            n178 = local write "Test Name"(u16 0) -> ()
          }
        }
      }
      event "Test Tree": Value Change {
        # "Show appropriate\ncontrols"
        n179 = event-data() -> ("CtlRef"=w327:refnum<vi>, "NewVal"=w325:string)  [unwired: 1 in]
        n180 = call <vilib>:"WPI_UtilitiesGetTreeIOName.vi"("NewVal"=w325, "TreeControl in"=w327) -> ("I/O Name"=w328:string)  [unwired: 9 in]
        n181 = case shown="\"Camera\"" w328 {
          selector: w328 -> [_ w335 _ w353 w362 _]
          tunnel: w325 -> [_ _ w350 w352 _ w369]
          tunnel: w324 -> [_ _ _ _ _ w368]
          frame Default {
            w330 = FALSE ("Visible")
            w329 = FALSE ("Visible")
            n182 = property on="Motor" class="Clust (strict)"("Visible"=w329) -> ()  [unwired: 2 in, 2 out]
            n183 = property on="Ring" class="Ring (strict)"("Visible"=w329) -> ()  [unwired: 2 in, 2 out]
            n184 = property on="Rev/Fwd" class="Clust (strict)"("Visible"=w330) -> ()  [unwired: 2 in, 2 out]
            n185 = property on="What is this?" class="Bool (strict)"("Visible"=w330) -> ()  [unwired: 2 in, 2 out]
            n186 = property on="Slider" class="Slide (strict)"("Visible"=w330) -> ()  [unwired: 2 in, 2 out]
          }
          frame "Motor", "PWM" {
            w336 = FALSE ("Visible")
            n187 = case shown="\"Motor\", Default" w335 {
              tunnel: [1.0 ("Value") -1.0 ("Value")] -> w334
              tunnel: [255.0 ("Value") 1.0 ("Value")] -> w333
              tunnel: [128.0 ("Value") 0.0 ("Value")] -> w332
              tunnel: [64.0 ("Value") 0.5 ("Value")] -> w331
              frame "PWM" {
              }
              frame "Motor", Default {
              }
            }
            n188 = property on="Motor" class="Clust (strict)"("Visible"=TRUE) -> ()  [unwired: 2 in, 2 out]
            n189 = property on="Value" class="Slide (strict)"("Value"=w332, "Scale.Minimum"=w334, "Scale.Maximum"=w333, "Scale.Increment"=w331) -> ()  [unwired: 2 in, 2 out]
            n190 = property on="What is this?" class="Bool (strict)"("Visible"=w336) -> ()  [unwired: 2 in, 2 out]
            n191 = property on="Slider" class="Slide (strict)"("Visible"=w336) -> ()  [unwired: 2 in, 2 out]
            n192 = property on="Ring" class="Ring (strict)"("Visible"=w336) -> ()  [unwired: 2 in, 2 out]
            n193 = property on="Rev/Fwd" class="Clust (strict)"("Visible"=w336) -> ()  [unwired: 2 in, 2 out]
          }
          frame "Servo" {
            w348 = FALSE ("Visible")
            n194 = call <vilib>:"NT Read Number.vi"("Name"=w350) -> ("Numeric"=w349:dbl)  [unwired: 9 in, 1 out]
            n195 = property on="Slider" class="Slide (strict)"("Visible"=TRUE, "Scale.Maximum"=170.0 ("Scale.Range:Maximum")) -> ()  [unwired: 2 in, 2 out]
            n196 = local write "Slider"(w349) -> ()
            n197 = property on="Motor" class="Clust (strict)"("Visible"=w348) -> ()  [unwired: 2 in, 2 out]
            n198 = property on="Rev/Fwd" class="Clust (strict)"("Visible"=w348) -> ()  [unwired: 2 in, 2 out]
            n199 = property on="What is this?" class="Bool (strict)"("Visible"=w348) -> ()  [unwired: 2 in, 2 out]
            n200 = property on="Ring" class="Ring (strict)"("Visible"=w348) -> ()  [unwired: 2 in, 2 out]
          }
          frame "Relay", "Solenoid" {
            w351 = FALSE ("Visible")
            n201 = property on="Motor" class="Clust (strict)"("Visible"=w351) -> ()  [unwired: 2 in, 2 out]
            n202 = property on="Slider" class="Slide (strict)"("Visible"=w351) -> ()  [unwired: 2 in, 2 out]
            n203 = Search and Replace String(input string=w352, search string="/Value  **", replace string="/Direction") -> (result string=w358:string)  [unwired: 5 in, 3 out]
            n204 = property on="Ring" class="Ring (strict)"("Visible"=w351) -> ()  [unwired: 2 in, 2 out]
            n205 = call <vilib>:"NT Read String.vi"("Name"=w358) -> ("String"=w356:string)  [unwired: 9 in, 1 out]
            n206 = Equal?(x="Both directions", y=w356) -> (x = y?=w354:bool)
            n207 = Not(x=w354) -> (.not. x?=w355:bool)
            n208 = property on="Rev/Fwd" class="Clust (strict)"("Visible"=w354) -> ()  [unwired: 2 in, 2 out]
            n209 = property on="What is this?" class="Bool (strict)"("Visible"=w355, "Caption.Text"=w353) -> ()  [unwired: 2 in, 2 out]
          }
          frame "Compressor", "Digital Out" {
            w361 = FALSE ("Visible")
            # "Get direction and finish"
            n210 = property on="Motor" class="Clust (strict)"("Visible"=w361) -> ()  [unwired: 2 in, 2 out]
            n211 = property on="Slider" class="Slide (strict)"("Visible"=w361) -> ()  [unwired: 2 in, 2 out]
            n212 = property on="Ring" class="Ring (strict)"("Visible"=w361) -> ()  [unwired: 2 in, 2 out]
            n213 = property on="What is this?" class="Bool (strict)"("Visible"=TRUE, "Caption.Text"=w362) -> ()  [unwired: 2 in, 2 out]
            n214 = property on="Rev/Fwd" class="Clust (strict)"("Visible"=FALSE) -> ()  [unwired: 2 in, 2 out]
          }
          frame "Camera" {
            n215 = call <vilib>:"Get Last Path Segment.vi"("String in"=w369) -> ("String out"=w370:string)  [unwired: 10 in]
            n216 = property on="What is this?" class="Bool (strict)"("Visible"=FALSE) -> ()  [unwired: 2 in, 2 out]
            n217 = property on="Motor" class="Clust (strict)"("Visible"=FALSE) -> ()  [unwired: 2 in, 2 out]
            n218 = property on="Rev/Fwd" class="Clust (strict)"("Visible"=FALSE) -> ()  [unwired: 2 in, 2 out]
            n219 = case shown="\"Exposure  **\"" w370 {
              tunnel: w369 -> [w376 w385 w394 w403 w412 _ w418]
              tunnel: w368 -> [w374 w382 w391 w400 w409 _ _]
              frame "Size  **" {
                n220 = Index Array(array=w374) -> (element=w373:cluster{string[]})  [unwired: 1 in]
                n221 = call <vilib>:"NT Read String.vi"("Name"=w376) -> ("String"=w375:string)  [unwired: 9 in, 1 out]
                n222 = Unbundle(w373) -> (w371:string[])
                n223 = Match First String(2:w371, 3:w375) -> (0:w372:i32)  [unwired: 1 out]
                n224 = property on="Ring" class="Ring (strict)"("Value"=w372, "Strings []"=w371) -> ()  [unwired: 2 in, 2 out]
                n225 = property on="Ring" class="Ring (strict)"("Visible"=TRUE) -> ()  [unwired: 2 in, 2 out]
                n226 = property on="Slider" class="Slide (strict)"("Visible"=FALSE) -> ()  [unwired: 2 in, 2 out]
              }
              frame "White Balance  **" {
                n227 = Index Array(array=w382, index=1) -> (element=w383:cluster{string[]})
                n228 = call <vilib>:"NT Read String.vi"("Name"=w385) -> ("String"=w384:string)  [unwired: 9 in, 1 out]
                n229 = Unbundle(w383) -> (w380:string[])
                n230 = Match First String(2:w380, 3:w384) -> (0:w379:i32)  [unwired: 1 out]
                n231 = property on="Ring" class="Ring (strict)"("Value"=w379, "Strings []"=w380) -> ()  [unwired: 2 in, 2 out]
                n232 = property on="Ring" class="Ring (strict)"("Visible"=TRUE) -> ()  [unwired: 2 in, 2 out]
                n233 = property on="Slider" class="Slide (strict)"("Visible"=FALSE) -> ()  [unwired: 2 in, 2 out]
              }
              frame "Exposure  **" {
                n234 = Index Array(array=w391, index=2) -> (element=w392:cluster{string[]})
                n235 = call <vilib>:"NT Read String.vi"("Name"=w394) -> ("String"=w393:string)  [unwired: 9 in, 1 out]
                n236 = Unbundle(w392) -> (w388:string[])
                n237 = Match First String(2:w388, 3:w393) -> (0:w389:i32)  [unwired: 1 out]
                n238 = property on="Ring" class="Ring (strict)"("Value"=w389, "Strings []"=w388) -> ()  [unwired: 2 in, 2 out]
                n239 = property on="Ring" class="Ring (strict)"("Visible"=TRUE) -> ()  [unwired: 2 in, 2 out]
                n240 = property on="Slider" class="Slide (strict)"("Visible"=FALSE) -> ()  [unwired: 2 in, 2 out]
              }
              frame "Exposure Priority  **" {
                n241 = Index Array(array=w400, index=3) -> (element=w401:cluster{string[]})
                n242 = call <vilib>:"NT Read String.vi"("Name"=w403) -> ("String"=w402:string)  [unwired: 9 in, 1 out]
                n243 = Unbundle(w401) -> (w397:string[])
                n244 = Match First String(2:w397, 3:w402) -> (0:w398:i32)  [unwired: 1 out]
                n245 = property on="Ring" class="Ring (strict)"("Value"=w398, "Strings []"=w397) -> ()  [unwired: 2 in, 2 out]
                n246 = property on="Ring" class="Ring (strict)"("Visible"=TRUE) -> ()  [unwired: 2 in, 2 out]
                n247 = property on="Slider" class="Slide (strict)"("Visible"=FALSE) -> ()  [unwired: 2 in, 2 out]
              }
              frame "Color Enable  **" {
                n248 = Index Array(array=w409, index=4) -> (element=w410:cluster{string[]})
                n249 = call <vilib>:"NT Read String.vi"("Name"=w412) -> ("String"=w411:string)  [unwired: 9 in, 1 out]
                n250 = Unbundle(w410) -> (w406:string[])
                n251 = Match First String(2:w406, 3:w411) -> (0:w407:i32)  [unwired: 1 out]
                n252 = property on="Ring" class="Ring (strict)"("Value"=w407, "Strings []"=w406) -> ()  [unwired: 2 in, 2 out]
                n253 = property on="Ring" class="Ring (strict)"("Visible"=TRUE) -> ()  [unwired: 2 in, 2 out]
                n254 = property on="Slider" class="Slide (strict)"("Visible"=FALSE) -> ()  [unwired: 2 in, 2 out]
              }
              frame Default {
                n255 = property on="Ring" class="Ring (strict)"("Visible"=FALSE) -> ()  [unwired: 2 in, 2 out]
                n256 = property on="Slider" class="Slide (strict)"("Visible"=FALSE) -> ()  [unwired: 2 in, 2 out]
              }
              frame "Brightness  **", "Color Level  **", "Compression  **", "FPS  **", "Sharpness  **" {
                n257 = call <vilib>:"NT Read Number.vi"("Name"=w418) -> ("Numeric"=w417:dbl)  [unwired: 9 in, 1 out]
                n258 = local write "Slider"(w417) -> ()
                n259 = property on="Slider" class="Slide (strict)"("Visible"=TRUE, "Scale.Maximum"=100.0 ("Scale.Range:Maximum")) -> ()  [unwired: 2 in, 2 out]
                n260 = property on="Ring" class="Ring (strict)"("Visible"=FALSE) -> ()  [unwired: 2 in, 2 out]
              }
            }
          }
        }
        n261 = property on="Progress" class="Clust (strict)"("Visible"=FALSE) -> ()  [unwired: 2 in, 2 out]
      }
      event "Test Name": Mouse Enter {
        # "Populate the ring with the list of tests"
        n262 = event-data() -> ()  [unwired: 1 in, 1 out]
        n263 = call <vilib>:"NT Read String Array.vi"("Name"="TestMode/TestList") -> ("String Array"=w425:string[])  [unwired: 9 in, 1 out]
        n264 = Build Array (concatenate)("Select the test to run...", w425) -> (w424:string[])
        n265 = property on="Test Name" class="Ring (strict)"("Strings []"=w424) -> ()  [unwired: 2 in, 2 out]
      }
      event "Test Name": Value Change {
        w427 = FALSE ("Visible")
        # "Tell the robot the test name to run"
        n266 = event-data() -> ("NewVal"=w431:u16)  [unwired: 1 in]
        n267 = property on="Test Name" class="Ring (strict)"() -> ("Strings []"=w432:string[])  [unwired: 2 in, 2 out]
        n268 = local write "Progress"(T4 {"Test Progress"=0, "Test Progress Text"=""} ("Progress")) -> ()
        n269 = Index Array(array=w432, index=w431) -> (element=w430:string)
        n270 = call <vilib>:"NT Write String.vi"("String"=w430, "Name"="TestMode/TestName") -> ()  [unwired: 9 in, 1 out]
        n271 = property on="Progress" class="Clust (strict)"("Visible"=TRUE) -> ()  [unwired: 2 in, 2 out]
        n272 = property on="Motor" class="Clust (strict)"("Visible"=w427) -> ()  [unwired: 2 in, 2 out]
        n273 = property on="Slider" class="Slide (strict)"("Visible"=w427) -> ()  [unwired: 2 in, 2 out]
        n274 = property on="What is this?" class="Bool (strict)"("Visible"=w427) -> ()  [unwired: 2 in, 2 out]
        n275 = property on="Rev/Fwd" class="Clust (strict)"("Visible"=w427) -> ()  [unwired: 2 in, 2 out]
        n276 = property on="Ring" class="Ring (strict)"("Visible"=w427) -> ()  [unwired: 2 in, 2 out]
      }
      event "Listbox": Double Click {
        n277 = event-data() -> ("PlatMods.Shift"=w435:bool, "Row"=w437:i32)  [unwired: 1 in]
        n278 = case shown="False" w435 {
          tunnel: w437 -> [w441 _]
          tunnel: 1 -> [w440 _]
          frame False {
            n279 = property on="Listbox" class="LstBox (strict)"() -> ("Item Symbols"=w439:i32[])  [unwired: 2 in, 2 out]
            n280 = Replace Array Subset(array=w439, new element=w440, index=w441) -> (w438:i32[])
            n281 = property on="Listbox" class="LstBox (strict)"("Item Symbols"=w438) -> ()  [unwired: 2 in, 2 out]
          }
          frame True {
            w442 = 0 ("Top Row")
            n282 = property on="Listbox" class="LstBox (strict)"() -> ("Number of Rows"=w444:u32)  [unwired: 2 in, 2 out]
            n283 = Initialize Array(0, w444) -> (w443:i32[])
            n284 = property on="Listbox" class="LstBox (strict)"("Top Row"=w442, "Value"=w442, "Item Symbols"=w443) -> ()  [unwired: 2 in, 2 out]
          }
        }
      }
      event "Listbox": Key Down {
        n285 = event-data() -> ("VKey"=w448:T18)  [unwired: 1 in]
        n286 = case shown="\"Left\", \"Right\"" w448 {
          selector: w448 -> [w453 _]
          tunnel: eventvkey."Left" ("VKey") -> [w451 _]
          frame "Left", "Right" {
            n287 = Equal?(x=w451, y=w453) -> (x = y?=w452:bool)
            n288 = Select(t=0, s=w452, f=1) -> (s? t:f=w454:i32)
            n289 = property on="Listbox" class="LstBox (strict)"() -> ("Item Symbols"=w457:i32[])  [unwired: 2 in, 2 out]
            n290 = Replace Array Subset(array=w457, new element=w454, index="Listbox") -> (w456:i32[])
            n291 = property on="Listbox" class="LstBox (strict)"("Item Symbols"=w456) -> ()  [unwired: 2 in, 2 out]
          }
          frame Default {
          }
        }
      }
      event "Low Cam Conf": Value Change {
        n292 = event-data() -> ("NewVal"=w461:bool)  [unwired: 1 in]
        n293 = case shown="False" w461 {
          tunnel: w460 -> [w470 _]
          tunnel: [w463 w481] -> w459
          tunnel: w458 -> [w462 w481]
          frame False {
            w477 = "LowCamera"
            w480 = FALSE ("Visible")
            n294 = local read "Low Camera Settings"() -> (w469:T1)
            n295 = Index Array(array=w470) -> (element=w473:cluster{string[]})  [unwired: 1 in]
            n296 = Unbundle(w469) -> ("Frate Rate"=w468:i32, "Compression"=w467:i32, "Size"=w471:u16)
            n297 = Unbundle(w473) -> (w472:string[])
            n298 = Index Array(array=w472, index=w471) -> (element=w466:string)
            n299 = call-poly <vilib>:"Write Key.vi"("section"=w477, "value"=w466, "key"="Size", "refnum"=w462) -> ("refnum out"=w479:T17)  [unwired: 2 in, 5 out]
            n300 = call-poly <vilib>:"Write Key.vi"("section"=w477, "value"=w468, "key"="FrameRate", "refnum"=w479) -> ("refnum out"=w478:T17)  [unwired: 1 in, 6 out]
            n301 = property on="Low Camera Settings" class="Clust (strict)"("Visible"=w480) -> ()  [unwired: 2 in, 2 out]
            n302 = local write "Low Cam Conf"(w480) -> ()
            n303 = call-poly <vilib>:"Write Key.vi"("section"=w477, "value"=w467, "key"="Compression", "refnum"=w478) -> ("refnum out"=w464:T17)  [unwired: 1 in, 6 out]
            n304 = call <vilib>:"Close Config Data.vi"("refnum"=w464) -> ("file path"=w465:path)  [unwired: 2 in, 8 out]
            n305 = call <vilib>:"Open Config Data.vi"("configuration file path"=w465) -> ("refnum"=w463:T17)  [unwired: 8 in, 2 out]
          }
          frame True {
            n306 = property on="Low Camera Settings" class="Clust (strict)"("Visible"=TRUE) -> ()  [unwired: 2 in, 2 out]
          }
        }
      }
      event "upper limit", "lower limit": Value Change {
        w487 = "Limits" ("section")
        n307 = event-data() -> ()  [unwired: 1 in, 1 out]
        n308 = local read "upper limit"() -> (w484:dbl)
        n309 = local read "lower limit"() -> (w483:dbl)
        n310 = call-poly <vilib>:"Write Key.vi"("section"=w487, "value"=w484, "key"="Upper", "refnum"=w492) -> ("refnum out"=w491:T17)  [unwired: 4 in, 3 out]
        n311 = call-poly <vilib>:"Write Key.vi"("section"=w487, "value"=w483, "key"="Lower", "refnum"=w491) -> ("refnum out"=w490:T17)  [unwired: 4 in, 3 out]
        n312 = call <vilib>:"Close Config Data.vi"("refnum"=w490) -> ("file path"=w489:path)  [unwired: 2 in, 8 out]
        n313 = call <vilib>:"Open Config Data.vi"("configuration file path"=w489) -> ("refnum"=w488:T17)  [unwired: 8 in, 2 out]
      }
      event "Low Camera Settings": Value Change {
        n314 = event-data() -> ("NewVal"=w504:T1)  [unwired: 1 in]
        n315 = Index Array(array=w500) -> (element=w499:cluster{string[]})  [unwired: 1 in]
        n316 = Unbundle(w504) -> ("Frate Rate"=w495:i32, "Compression"=w494:i32, "Size"=w497:u16)
        n317 = Unbundle(w499) -> (w498:string[])
        n318 = Index Array(array=w498, index=w497) -> (element=w496:string)
        n319 = Format Into String(format string="%s   %dfps   %d%%", w496, w495, w494) -> (resulting string=w501:string)  [unwired: 2 in, 1 out]
        n320 = Build Array(w501) -> (w502:string[])
        n321 = property on="Low Cam Conf" class="Bool (strict)"("Strings [4]"=w502) -> ()  [unwired: 2 in, 2 out]
      }
      event "Motor.Enable": Value Change {
        n322 = event-data() -> ("NewVal"=w510:bool)  [unwired: 1 in]
        n323 = Unbundle("Motor") -> ("Value"=w509:dbl)  [unwired: 1 out]
        n324 = Select(t=w509, s=w510, f=0.0) -> (s? t:f=w507:dbl)
        n325 = call <vilib>:"NT Write Number.vi"("Numeric"=w507, "Name"=w506) -> ()  [unwired: 9 in, 1 out]
      }
      event "Slider": Value Change {
        n326 = event-data() -> ("NewVal"=w513:dbl)  [unwired: 1 in]
        n327 = call <vilib>:"NT Write Number.vi"("Numeric"=w513, "Name"=w514) -> ()  [unwired: 9 in, 1 out]
      }
      event "What is this?": Value Change {
        n328 = event-data() -> ("NewVal"=w518:bool)  [unwired: 1 in]
        n329 = Boolean To (0,1)(Boolean=w518) -> (0, 1=w517:i16)
        n330 = call <vilib>:"NT Write Number.vi"("Numeric"=w517, "Name"=w516) -> ()  [unwired: 9 in, 1 out]
      }
      event "CaptureScreen": Value Change {
        n331 = event-data() -> ()  [unwired: 1 in, 1 out]
        n332 = flat-sequence {
          tunnel: [FALSE ("CaptureScreen")] -> w519
          tunnel: w519 -> [w531]
          frame #0 {
            n333 = local read "Camera Image Diag"() -> (w529:T2)
            n334 = local read "Low Camera Image"() -> (w530:T2)
            n335 = local read "Processed Image"() -> (w528:T2)
            n336 = Build Array(w530, w529, w528) -> (w524:T2[])
            n337 = Build Array("_enhanced.jpg", "_raw.jpg", "_vision.jpg") -> (w522:string[])
            n338 = Wait (ms)(milliseconds to wait=u32 200) -> ()  [unwired: 1 out]
            n339 = call "BB_Take Screenshots.vi"("Image_Labels"=w522, "Prefix"="Filename", "Image_Array"=w524) -> ()  [unwired: 8 in, 1 out]
          }
          frame #1 {
            n340 = property on="CaptureScreen" class="Bool (strict)"("Value"=w531) -> ()  [unwired: 2 in, 2 out]
          }
        }
      }
      event "Rev/Fwd": Value Change {
        n341 = event-data() -> ("NewVal.Forward"=w539:bool, "NewVal.Reverse"=w538:bool)  [unwired: 1 in]
        n342 = Boolean To (0,1)(Boolean=w539) -> (0, 1=w535:i16)
        n343 = Boolean To (0,1)(Boolean=w538) -> (0, 1=w537:i16)
        n344 = Negate(x=w537) -> (-x=w536:i16)
        n345 = Add(x=w535, y=w536) -> (x+y=w534:i16)
        n346 = call <vilib>:"NT Write Number.vi"("Numeric"=w534, "Name"=w533) -> ()  [unwired: 9 in, 1 out]
      }
      event "Ring": Value Change {
        n347 = event-data() -> ("NewVal"=w543:u16)  [unwired: 1 in]
        n348 = property on="Ring" class="Ring (strict)"() -> ("Strings []"=w544:string[])  [unwired: 2 in, 2 out]
        n349 = Index Array(array=w544, index=w543) -> (element=w542:string)
        n350 = call <vilib>:"NT Write String.vi"("String"=w542, "Name"=w541) -> ()  [unwired: 9 in, 1 out]
      }
    }
  }
  n351 = call "IMAQ Create"("Image Name"="Destination", "Image Type"=w31) -> ("New Image"=w29:T2)  [unwired: 2 in, 2 out]
  n352 = while {
    tunnel: [w570] -> _
    tunnel: w29 -> [w563]
    tunnel: w27 -> [w561]
    tunnel: w26 -> [w558]
    tunnel: w23 -> [w551]
    i -> [w570]
    stop <- FALSE stop-if-true
    n353 = local read "Low Camera Settings"() -> (w560:T1)
    n354 = global write "Angle.vi" "Camera view angle"("Camera view angle") -> ()
    n355 = call "BB_CameraSet Brightness.vi"("Brightness"="Low Brightness", "Camera Address"=w561) -> ("error out"=w557:errorcluster, "Camera Address Out"=w559:string)  [unwired: 8 in]
    n356 = call <vilib>:"WPI_CameraRead MJPG.vi"("error in"=w557, "Camera Settings"=w560, "Image"=w558, "address"=w559) -> ("error out"=w552:errorcluster, "Bandwidth (kbps)"=w553:dbl, "Image Out"=w547:T2)  [unwired: 5 in]
    "L Mbps" <- w553
    n357 = call "IMAQ ColorBCGLookup"("error in (no error)"=w552, "Image Dst"=w551, "Image Src"=w547) -> ("error out"=w548:errorcluster, "Image Dst Out"=w549:T2)  [unwired: 7 in]
    n358 = call "BB_Draw_rect.vi"("Error In"=w548, "Image In"=w549) -> ("Error Out"=w545:errorcluster, "Image"=→"Low Camera Image":T2)  [unwired: 8 in]
    n359 = Unbundle("Low Camera Settings") -> ("Frate Rate"=w554:i32)  [unwired: 2 out]
    n360 = Unbundle By Name(w545) -> ("status"=w546:bool)
    n361 = call "FPS Calculator.vi"("Average Count"=w554) -> ("fps"=→"L_FPS":dbl)  [unwired: 10 in]
    n362 = property on="Image Error Message" class="Str"("Visible"=w546) -> ()  [unwired: 2 in, 2 out]
    n363 = Unbundle(w545) -> ("status"=w569:bool)  [unwired: 2 out]
    n364 = Compound Arithmetic op=AND(TRUE, invert w569) -> (w568:bool)
    n365 = case shown="True" w568 {
      tunnel: w547 -> [_ w587]
      tunnel: w553 -> [_ w586]
      tunnel: "Low Dilate_its" -> [_ w584]
      tunnel: "Low Erode_its" -> [_ w583]
      tunnel: w563 -> [_ w574]
      frame False {
        n366 = Wait Until Next ms Multiple(millisecond multiple=u32 30) -> ()  [unwired: 1 out]
      }
      frame True {
        # "Display image and save\nthe occasional frame to disk.\nThe image can also be processed here."
        # "Update Mbps\nindicator"
        n367 = call "IMAQ Clear Overlay"("Image"=w587) -> ("Image Out"=w575:T2)  [unwired: 2 in, 8 out]
        "Camera Image Diag" <- w575
        n368 = case shown="Default" w586 {
          tunnel: [u32 6618880 ("Color Box") u32 16776722 ("Color Box") u32 16716800 ("Color Box")] -> w588
          frame Default {
          }
          frame 4, 5 {
          }
          frame 6.. {
          }
        }
        n369 = Bundle("Color Box"=w588, "Color Box"=w588) -> (w590:cluster{"Color Box":u32, "Color Box":u32})  [unwired: 1 out]
        n370 = Build Array(w590) -> (w589:cluster{"Color Box":u32, "Color Box":u32}[])
        n371 = property on="BW" class="Bool (strict)"("Colors [4]"=w589) -> ()  [unwired: 2 in, 2 out]
        n372 = call "Save DB Images.vi"("Images to Keep"=600.0, "Image"=w575) -> ()  [unwired: 1 in, 1 out]
        n373 = call "Vision Proc (SubVI).vi"("Image In"=w575, "Dilate_its"=w584, "Image Dst"=w574, "Erode_its"=w583, "Annotate"=TRUE) -> ("Processed Image"=→"Processed Image":T2, "Target Info"=w582:T7)  [unwired: 18 in, 3 out]
        "Target Info" <- w582
        n374 = call "sendCenterTarget.vi"("Target Info"=w582) -> ("Values"=w581:T8)  [unwired: 10 in]
        "Values" <- w581
        n375 = Unbundle By Name(w581) -> ("distanceToCenter"=w580:dbl, "angleToCenter"=w578:dbl)
        n376 = call "Moving Average.vi"("Numeric in"=w580) -> ("Numeric out"=→"Range to Center":dbl)  [unwired: 10 in]
        n377 = call "Moving Average.vi"("Numeric in"=w578) -> ("Numeric out"=→"Angle to Center":dbl)  [unwired: 10 in]
      }
    }
  }
  n378 = while {
    stop <- FALSE stop-if-true
    # "File Transfer"
    n379 = local read "Robot IP"() -> (w595:string)
    n380 = event shown="[0] Timeout" {
      selector: _ -> [_ _ _ _ _ _ _]
      dyn-events: _ -> [_ _ _ _ _ _ _]
      timeout: 100 -> [_ _ _ _ _ _ _]
      tunnel: "working directory" -> [_ w598 w602 w606 w627 w648 w656]
      tunnel: w595 -> [_ _ _ w607 w628 _ w655]
      event Timeout {
        n381 = event-data() -> ()  [unwired: 1 in, 2 out]
      }
      event "Edit Vision Distance Table CSV": Value Change {
        n382 = event-data() -> ()  [unwired: 1 in, 5 out]
        n383 = call "Open Excel Report.vi"("Filename"="2013VisionTable.csv" ("command line"), "Base Path"=w598) -> ("error out"=w600:errorcluster)  [unwired: 9 in]
        n384 = Unbundle By Name(w600) -> ("source"=w599:string)
        n385 = local write "standard output"(w599) -> ()
      }
      event "Edit Autonomous CSV": Value Change {
        n386 = event-data() -> ()  [unwired: 1 in, 5 out]
        n387 = call "Open Excel Report.vi"("Filename"="2013AutoModesJava.csv" ("command line"), "Base Path"=w602) -> ("error out"=w604:errorcluster)  [unwired: 9 in]
        n388 = Unbundle By Name(w604) -> ("source"=w603:string)
        n389 = local write "standard output"(w603) -> ()
      }
      event "Transfer Vision Distance Table  to cRIO": Value Change {
        w615 = ""
        w614 = "anonymous"
        w613 = "/2013VisionTable.csv"
        n390 = event-data() -> ()  [unwired: 1 in, 5 out]
        n391 = Build Path(base path=w606, name or relative path="2013VisionTableLast.csv") -> (appended path=w616:path)
        n392 = call <vilib>:"FTP Get File.vi"("active (T)"=FALSE, "password"=w615, "binary (F)"=TRUE, "user"=w614, "local path"=w616, "remote path"=w613, "host"=w607) -> ("error out"=w621:errorcluster)  [unwired: 3 in, 1 out]
        n393 = case shown="Error" w621 {
          tunnel: ["Saved Last" "Save Failed"] -> w622
          frame No Error {
          }
          frame Error {
          }
        }
        "standard output" <- w622
        n394 = Build Path(base path=w606, name or relative path="2013VisionTable.csv") -> (appended path=w617:path)
        n395 = call <vilib>:"FTP Put File.vi"("active (T)"=FALSE, "password"=w615, "binary (F)"=TRUE, "user"=w614, "error in (no error)"=w621, "local path"=w617, "remote path"=w613, "host"=w607) -> ("file error"=w619:errorcluster)  [unwired: 2 in, 1 out]
        n396 = case shown="Error" w619 {
          tunnel: ["Successfully Completed" "Transfer Failed"] -> w620
          frame No Error {
          }
          frame Error {
          }
        }
        n397 = local write "standard output"(w620) -> ()
      }
      event "Transfer Autonomous CSV to cRIO": Value Change {
        w636 = ""
        w637 = "anonymous"
        w638 = "/2013AutoModesJava.csv"
        n398 = event-data() -> ()  [unwired: 1 in, 5 out]
        n399 = Build Path(base path=w627, name or relative path="2013AutoModesJavaLast.csv") -> (appended path=w635:path)
        n400 = call <vilib>:"FTP Get File.vi"("active (T)"=FALSE, "password"=w636, "binary (F)"=TRUE, "user"=w637, "local path"=w635, "remote path"=w638, "host"=w628) -> ("error out"=w630:errorcluster)  [unwired: 3 in, 1 out]
        n401 = case shown="No Error" w630 {
          tunnel: ["Saved Last" "Save Failed"] -> w629
          frame No Error {
          }
          frame Error {
          }
        }
        "standard output" <- w629
        n402 = Build Path(base path=w627, name or relative path="2013AutoModesJava.csv") -> (appended path=w634:path)
        n403 = call <vilib>:"FTP Put File.vi"("active (T)"=FALSE, "password"=w636, "binary (F)"=TRUE, "user"=w637, "error in (no error)"=w630, "local path"=w634, "remote path"=w638, "host"=w628) -> ("file error"=w632:errorcluster)  [unwired: 2 in, 1 out]
        n404 = case shown="Error" w632 {
          tunnel: ["Successfully Completed" "Transfer Failed"] -> w631
          frame No Error {
          }
          frame Error {
          }
        }
        n405 = local write "standard output"(w631) -> ()
      }
      event "Open Auto Commands Doc": Value Change {
        n406 = event-data() -> ()  [unwired: 1 in, 5 out]
        n407 = Build Path(base path=w648, name or relative path="BeachbotAutoCmdsDoc.html" ("command line")) -> (appended path=w653:path)
        n408 = Path To String(path=w653) -> (string=w651:string)
        n409 = Concatenate Strings("file:///", w651) -> (w650:string)
        n410 = call-poly <vilib>:"Open URL in Default Browser.vi"("URL"=w650) -> ("URL out"=w649:string)  [unwired: 5 in, 1 out]
        n411 = local write "standard output"(w649) -> ()
      }
      event "Transfer INI From cRIO": Value Change {
        n412 = event-data() -> ()  [unwired: 1 in, 5 out]
        n413 = Build Path(base path=w656, name or relative path="wpilib-preferences.ini") -> (appended path=w664:path)
        n414 = Build Path(base path=w656, name or relative path="wpilib-preferencesLast.ini") -> (appended path=w662:path)
        n415 = call <vilib>:"Check if File or Folder Exists.vi"("path"=w664) -> ("error out"=w666:errorcluster, "file or folder exists?"=w661:bool, "dup path"=w665:path)  [unwired: 8 in]
        n416 = Move(source path=w665, error in=w666, 9:w661, 10:w662) -> (error out=w660:errorcluster)  [unwired: 1 in, 2 out]
        n417 = case shown="No Error" w660 {
          tunnel: ["/nSaved Last" "/nSave Failed"] -> w659
          frame No Error {
          }
          frame Error {
          }
        }
        n418 = call <vilib>:"FTP Get File.vi"("active (T)"=FALSE, "password"="", "binary (F)"=TRUE, "user"="anonymous", "error in (no error)"=w660, "local path"=w664, "remote path"="/wpilib-preferences.ini", "host"=w655) -> ("error out"=w657:errorcluster)  [unwired: 2 in, 1 out]
        n419 = local write "standard output"(w659) -> ()
        n420 = case shown="Error" w657 {
          tunnel: ["Successfully Completed" "/nTransfer Failed"] -> w658
          frame No Error {
          }
          frame Error {
          }
        }
        n421 = local write "standard output"(w658) -> ()
      }
    }
  }
  n422 = flat-sequence {
    frame #0 {
      # "File Transfer GUI Controls"
      n423 = call <vilib>:"Application Directory.vi"() -> ("Application Directory"=w677:path)
      n424 = local write "working directory"(w677) -> ()
    }
  }
  n425 = property on="What is this?" class="Bool (strict)"("Visible"=w32) -> ()  [unwired: 2 in, 2 out]
  n426 = property on="Motor" class="Clust (strict)"("Visible"=w32) -> ()  [unwired: 2 in, 2 out]
  n427 = property on="Progress" class="Clust (strict)"("Visible"=w32) -> ()  [unwired: 2 in, 2 out]
  n428 = property on="Ring" class="Ring (strict)"("Visible"=w32) -> ()  [unwired: 2 in, 2 out]
  n429 = property on="Rev/Fwd" class="Clust (strict)"("Visible"=w32) -> ()  [unwired: 2 in, 2 out]
  n430 = local write "Low Cam Conf"(w32) -> ()
  n431 = local write "High Cam Conf"(w32) -> ()
  n432 = property on="Low Camera Settings" class="Clust (strict)"("Visible"=w32) -> ()  [unwired: 2 in, 2 out]
  n433 = flat-sequence {
    frame #0 {
      w678 = FALSE ("Visible")
      w679 = u32 1 items=["Grayscale", "Binary", "Gradient", "Rainbow", "Temperature", "User Defined"] ("Palette:Palette Type")
      # "User Interface"
      n434 = property on="String" class="Str"("Visible"=w678) -> ()  [unwired: 2 in, 2 out]
      n435 = property on="Number" class="DigNum (strict)"("Visible"=w678) -> ()  [unwired: 2 in, 2 out]
      n436 = property on="On/Off" class="Bool (strict)"("Visible"=w678) -> ()  [unwired: 2 in, 2 out]
      n437 = property on="Processed Image" class="ImageControl"("Palette Type"=w679) -> ()  [unwired: 2 in, 2 out]
    }
  }
  n438 = flat-sequence {
    frame #0 {
      # "Autonomous Mode Script Select"
      n439 = control-ref of="Autonomous\nMode"() -> (w681:refnum<vi>)
      n440 = call "DashboardSelectAuto.vi"("Table Prefix"="Autonomous mode", "Autonomous Mode Ring"=w681) -> ()  [unwired: 9 in]
    }
  }
